vi "Write FP Source Dir.vi"(5 "FP Source Dir":path=path "", 9 "RasPi Compiler in":refnum<class "RasPi Compiler.lvclass">) -> (3 "RasPi Compiler out":refnum<class "RasPi Compiler.lvclass">)   [LabVIEW 2014, in "RasPi Compiler.lvclass"]
uses:
  RasPi Compiler.lvclass
  RasPi Compiler.lvclass/RasPi Compiler.ctl
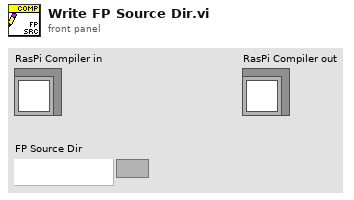
[diagram p1: front panel]
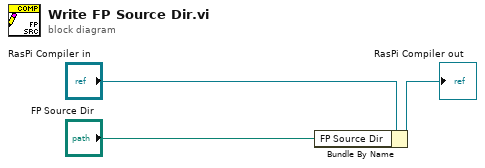
[diagram p0: block diagram]
diagram:
  n1 = Bundle By Name(cluster="RasPi Compiler in", "FP Source Dir"="FP Source Dir") -> (→"RasPi Compiler out":refnum<class "RasPi Compiler.lvclass">)
